vi "Read Config Handle.vi"(8 "error in":errorcluster, 11 "DAQ Device in":refnum<class "DAQ Device.lvclass">) -> (0 "error out":errorcluster, 2 "Session Handle":T1, 3 "DAQ Device out":refnum<class "DAQ Device.lvclass">)   [LabVIEW 2014, in "DAQ Device.lvclass"]
uses:
  DAQ Device.lvclass
  Session APIs/File Access/Config Data/Config Session.ctl
  Session APIs/File Access/Config Data/Config Data.lvclass
  DAQ Device.lvclass/DAQ Device.ctl
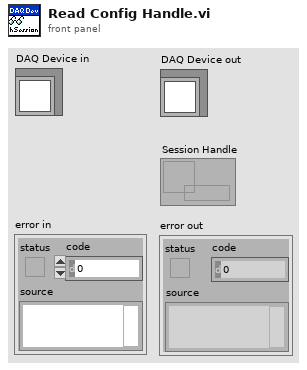
[diagram p1: front panel]
types:
  T1 = typedef "Config Data.lvclass/Config Session.ctl" = refnum<data-value>
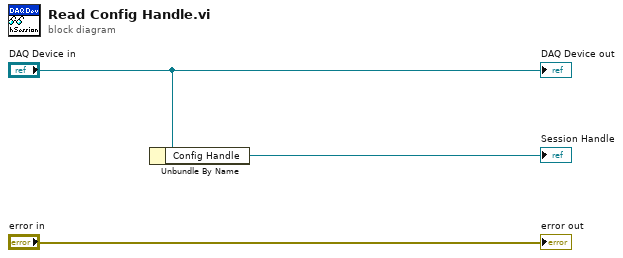
[diagram p0: block diagram]
diagram:
  n1 = Unbundle By Name("DAQ Device in") -> ("Config Handle"=→"Session Handle":T1)
  "error out" <- "error in"
  "DAQ Device out" <- "DAQ Device in"
